vi "Get Measurement Details.vi"(8 "error in":errorcluster) -> (0 "error out":errorcluster, 1 "Measurement Annotations":T1[](array[typedef])=[{"key"="", "value"=""}, {"key"="ni/service.collection", "value"="NI.Examples"}, {"key"="ni/service.tags", "value"="[]"}], 2 "Service Class":string, 3 "Measurement Details":T2)   [LabVIEW 2020, in "UIProgressUpdates.lvlib"]
uses:
  UIProgressUpdates.lvlib
  <vilib>/MeasurementLink/MeasurementLink Measurement Server/Helpers/TypeDefs/MeasurementDetails.ctl
  <vilib>/MeasurementLink/MeasurementLink Measurement Server/Helpers/TypeDefs/MeasurementAnnotation.ctl
  <vilib>/MeasurementLink/MeasurementLink Measurement Server/MeasurementLink Measurement Server.lvlib
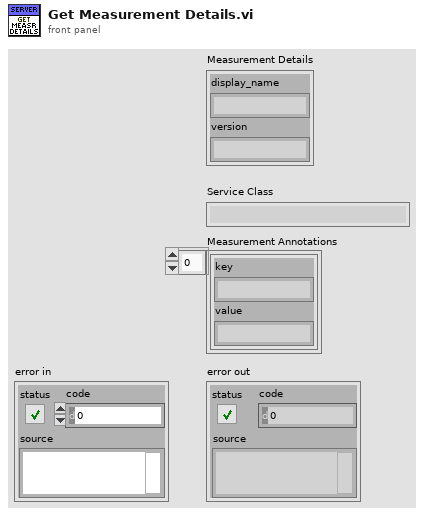
[diagram p1: front panel]
types:
  T1 = typedef "MeasurementLink Measurement Server.lvlib/MeasurementAnnotation.ctl" = cluster{"key":string, "value":string}
  T2 = typedef "MeasurementLink Measurement Server.lvlib/MeasurementDetails.ctl" = cluster{"display_name":string, "version":string}
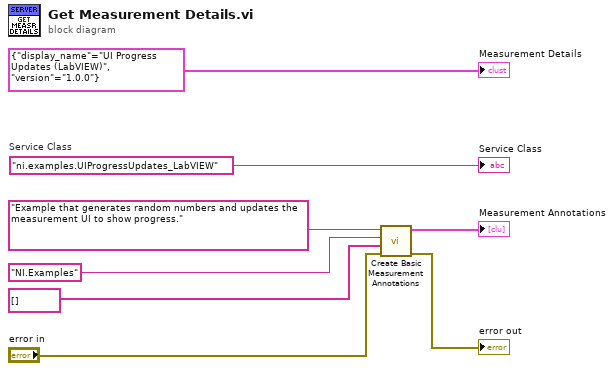
[diagram p0: block diagram]
diagram:
  w8 = "ni.examples.UIProgressUpdates_LabVIEW"  # Service Class
  n1 = call <vilib>:"Create Basic Measurement Annotations.vi"("error in"="error in", "Tags"=string[] [] ("ni/service.tags"), "Collection"="NI.Examples" ("ni/service.collection"), "Description"="Example that generates random numbers and updates the measurement UI to show progress." ("ni/service.description")) -> ("error out"=→"error out":errorcluster, "Measurement Annotations"=→"Measurement Annotations":T1[])  [unwired: 6 in]
  "Measurement Details" <- T2 {"display_name"="UI Progress Updates (LabVIEW)", "version"="1.0.0"} ("Measurement Details")
  "Service Class" <- w8
